vi "Lights Handler.vi"   [LabVIEW 2020]
uses:
  14d7c209-9479-431a-9046-3befd214614e.vi
  4911ac5a-636d-4ccd-96b5-939d6fc666c8.vi
  <vilib>/Rock Robotics/WPI/Utilities/WPI_GetSetVariantRefNum.vi
  Framework/Robot Global Data.vi
types:
  T1 = typedef "WPI_JoystickDevRef.ctl" = cluster{"Device":T2}
  T2 = typedef "WPI_JoystickDeviceEnum.ctl" = enum16{"USB 0", "USB 1", "USB 2", "USB 3", "USB 4", "USB 5"}
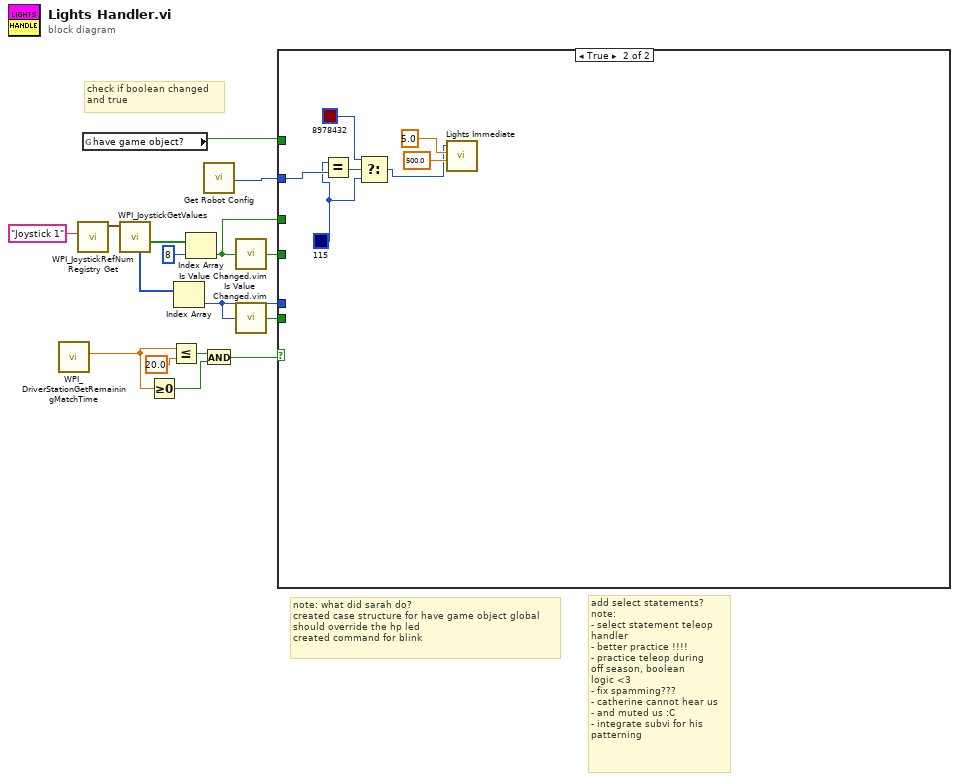
[diagram p0: block diagram]
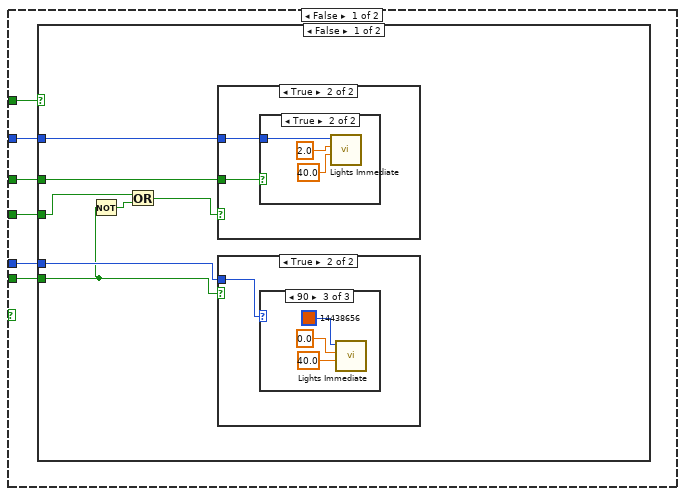
[diagram p2: hidden frame]
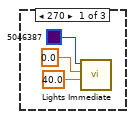
[diagram p6: hidden frame]
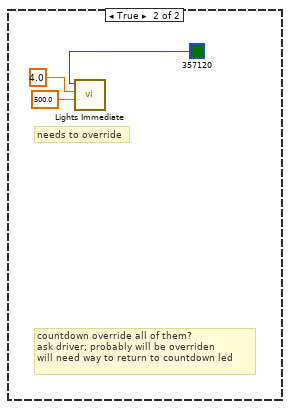
[diagram p8: hidden frame]
diagram:
  # "check if boolean changed\nand true"
  # "add select statements?\nnote: \n- select statement teleop \nhandler\n- better practice !!!! \n- practice teleop during\noff season, boolean \nlogic <3\n- fix spamming???\n- catherine cannot hear us\n- and muted us :C\n- integrate subvi for his \npatterning"
  # "note: what did sarah do?\ncreated case structure for have game object global\nshould override the hp led\ncreated command for blink"
  n1 = call <vilib>:"WPI_DriverStationGetRemainingMatchTime.vi"() -> ("Match Time(s)"=w3:sgl)  [unwired: 10 in, 1 out]
  n2 = call <vilib>:"WPI_JoystickRefNum Registry Get.vi"("refnum name"="Joystick 1") -> ("JoystickDevRef"=w15:T1)  [unwired: 1 in, 9 out]
  n3 = global read "Robot Global Data.vi" "have game object?"() -> (w2:bool)
  n4 = call <vilib>:"WPI_JoystickGetValues.vi"("JoystickDevRef"=w15) -> ("Buttons"=w12:bool[], "POVs"=w14:i16[])  [unwired: 6 in, 3 out]
  n5 = Greater Or Equal To 0?(x=w3) -> (x >= 0?=w1:bool)
  n6 = Less Or Equal?(x=w3, y=sgl 20.0) -> (x <= y?=w6:bool)
  n7 = Index Array(array=w14) -> (element=w8:i16)  [unwired: 1 in]
  n8 = Index Array(array=w12, index=8) -> (element=w4:bool)
  n9 = call "Get Robot Config.vi"() -> ("Color"=w7:u32)  [unwired: 12 in, 7 out]
  n10 = And(x=w6, y=w1) -> (x .and. y?=w5:bool)
  n11 = call "Is Value Changed.vim"("value"=w4) -> ("changed or first call?"=w10:bool)
  n12 = call "Is Value Changed.vim"("value"=w8) -> ("changed or first call?"=w9:bool)
  n13 = case shown="True" w5 {
    tunnel: w2 -> [w22 _]
    tunnel: w10 -> [w21 _]
    tunnel: w4 -> [w20 _]
    tunnel: w9 -> [w19 _]
    tunnel: w8 -> [w18 _]
    tunnel: w7 -> [w17 w48]
    frame False {
      n14 = case shown="False" w22 {
        tunnel: w21 -> [w24 _]
        tunnel: w20 -> [w26 _]
        tunnel: w19 -> [w25 _]
        tunnel: w18 -> [w29 _]
        tunnel: w17 -> [w28 _]
        frame False {
          n15 = Not(x=w25) -> (.not. x?=w27:bool)
          n16 = Or(x=w24, y=w27) -> (x .or. y?=w23:bool)
          n17 = case shown="True" w23 {
            tunnel: w26 -> [_ w31]
            tunnel: w28 -> [_ w30]
            frame False {
            }
            frame True {
              n18 = case shown="True" w31 {
                tunnel: w30 -> [_ w32]
                frame False {
                }
                frame True {
                  n19 = call "Lights Immediate.vi"("Speed"=40.0, "Flash Type"=2.0, "Color"=w32) -> ()  [unwired: 8 in, 1 out]
                }
              }
            }
          }
          n20 = case shown="True" w25 {
            tunnel: w29 -> [_ w35]
            frame False {
            }
            frame True {
              n21 = case shown="90" w35 {
                frame 270 {
                  n22 = call "Lights Immediate.vi"("Speed"=40.0, "Flash Type"=0.0, "Color"=u32 5046387 ("Purple")) -> ()  [unwired: 8 in, 1 out]
                }
                frame -1, Default {
                }
                frame 90 {
                  n23 = call "Lights Immediate.vi"("Speed"=40.0, "Flash Type"=0.0, "Color"=u32 14438656 ("Yellow")) -> ()  [unwired: 8 in, 1 out]
                }
              }
            }
          }
        }
        frame True {
          # "countdown override all of them?\nask driver; probably will be overriden\nwill need way to return to countdown led"
          # "needs to override"
          n24 = call "Lights Immediate.vi"("Speed"=500.0, "Flash Type"=4.0, "Color"=u32 357120 ("green")) -> ()  [unwired: 8 in, 1 out]
        }
      }
    }
    frame True {
      w46 = u32 115 ("Blue")
      n25 = Equal?(x=w46, y=w48) -> (x = y?=w47:bool)
      n26 = Select(t=u32 8978432 ("Red"), s=w47, f=w46) -> (s? t:f=w49:u32)
      n27 = call "Lights Immediate.vi"("Speed"=500.0, "Flash Type"=5.0, "Color"=w49) -> ()  [unwired: 8 in, 1 out]
    }
  }
